vi "CSM - Module Exit Event.vi"(8 "Error in":errorcluster caption="Error in (no error)", 11 "Name(\"\" to use uuid) in":string) -> (0 "Error out":errorcluster, 3 "CSM Exit Event":refnum<user-event>)   [LabVIEW 2020, in "Communicable State Machine.lvlib"]
doc: "Obtain CSM Global Log Event Reference.\n- <b>Error in</b>: Error cluster\n- <b>CSM Global Log Event</b>: User event reference for CSM global log.\n- <b>Error out</b>: Error cluster\n\n<b>Inputs:</b>\n - <b>Error in</b>:\n - <b>Name(\"\" to use uuid) in</b>:\n\n<b>Outputs:</b>\n - <b>Error out</b>:\n - <b>Status Change Event</b>:"
uses:
  Communicable State Machine.lvlib
  _CSMOFGVOPER.ctl
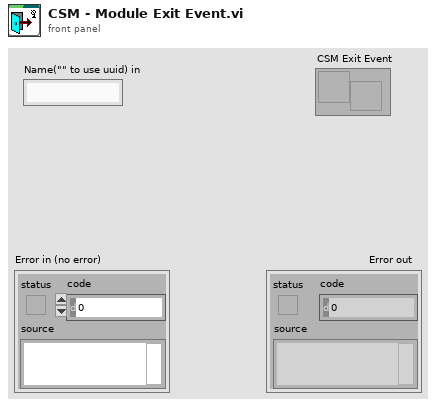
[diagram p1: front panel]
types:
  T1 = typedef "Communicable State Machine.lvlib/_CSMOFGVOPER.ctl" = enum16{"Create If not Exist", "Get By Name", "List", "Check If Name Exists", "Release", "Module Status", "Create Status Event Handler", "Destroy Status Event Handler"}
  T2 = typedef "Communicable State Machine.lvlib/_CSMObj.ctl" = cluster{"Requested Name":string, "Module Name":string, "Mode":T3, "Queue":refnum<class "Priority Queue.lvclass">, "CSM-Data":refnum<data-value>, "User Event":refnum<user-event>, "Status Change Event":refnum<user-event>, "Allowed Messages":string[], "Mode-Data":refnum<data-value>, "Group Name":string, "Exit Event":refnum<user-event>}
  T3 = typedef "Communicable State Machine.lvlib/_CSM_MODE.ctl" = enum16{"Not Exist", "Stand Alone", "CSM", "Worker Agent", "Worker", "Chain", "Chain Node"}
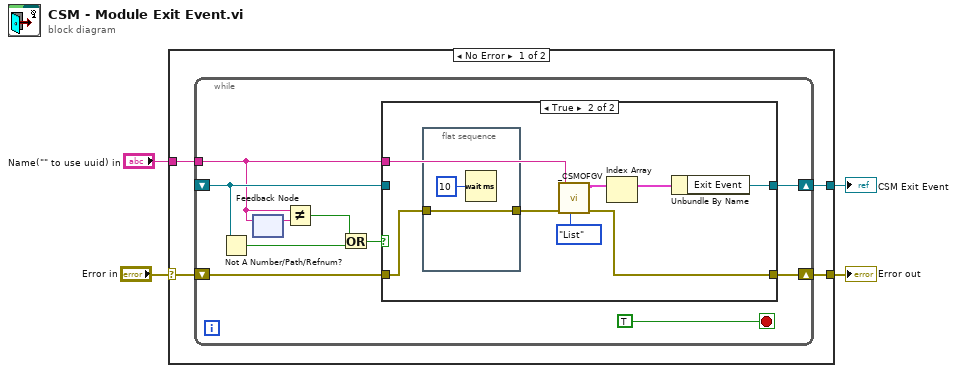
[diagram p0: block diagram]
diagram:
  n1 = case shown="No Error" "Error in" {
    selector: "Error in" -> [w7 w31]
    tunnel: [w8 _] -> w2
    tunnel: [w6 w31] -> w3
    tunnel: "Name(\"\" to use uuid) in" -> [w5 _]
    frame No Error {
      n2 = while {
        shift-right: [w16] -> w6
        shift-left: w7 -> [w17]
        shift-right: [w18] -> w8
        shift-left: _ -> [w14]
        tunnel: w5 -> [w12]
        stop <- TRUE stop-if-true
        n3 = Not A Number/Path/Refnum?(number/path/refnum=w14) -> (NaN/Path/Refnum?=w10:bool)
        n4 = feedback-in #1(w12) -> ()
        n5 = feedback #1() -> (w11:string)  [unwired: 1 in]
        n6 = Not Equal?(x=w12, y=w11) -> (x != y?=w9:bool)
        n7 = Or(x=w9, y=w10) -> (x .or. y?=w13:bool)
        n8 = case shown="True" w13 {
          tunnel: [w20 w24] -> w18
          tunnel: w17 -> [w19 w21]
          tunnel: [w19 w27] -> w16
          tunnel: w14 -> [w20 _]
          tunnel: w12 -> [_ w23]
          frame False {
          }
          frame True {
            n9 = flat-sequence {
              tunnel: [w29] -> w22
              tunnel: w21 -> [w29]
              frame #0 {
                n10 = Wait (ms)(milliseconds to wait=u32 10) -> ()  [unwired: 1 out]
              }
            }
            n11 = call "_CSMOFGV.vi"("Operation"=_CSMOFGVOPER."List", "Error in"=w22, "Name(\"\" to use uuid) in"=w23) -> ("Error out"=w27:errorcluster, "Array"=w26:T2[])  [unwired: 6 in, 1 out]
            n12 = Index Array(array=w26) -> (element=w25:T2)  [unwired: 1 in]
            n13 = Unbundle By Name(w25) -> ("Exit Event"=w24:refnum<user-event>)
          }
        }
      }
    }
    frame Error {
    }
  }
  "Error out" <- w3
  "CSM Exit Event" <- w2
